vi "Create.vi"(8 "error in (no error)":errorcluster, 9 "Calculation Period (ms)":u32=500, 10 "XNET Session":refnum<k21>, 11 "LINBus_Load_Calculator in":refnum<class "LINBus_Load_Calculator.lvclass">) -> (0 "error out":errorcluster, 3 "LINBus_Load_Calculator out":refnum<class "LINBus_Load_Calculator.lvclass">)   [LabVIEW 2019, in "XNET-Bus-Load-Calculator.lvlib" / "LINBus_Load_Calculator.lvclass"]
uses:
  LINBus_Load_Calculator.lvclass
  GenBus/GenBus_Load_Calculator.lvclass
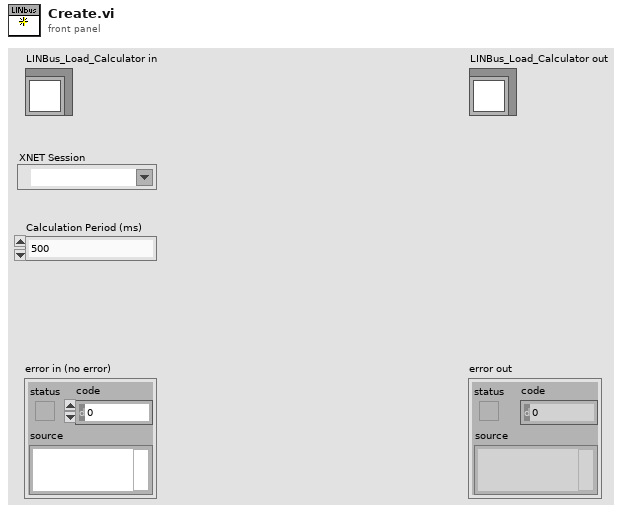
[diagram p1: front panel]
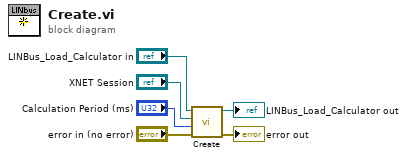
[diagram p0: block diagram]
diagram:
  n1 = call-parent "Create.vi"("error in (no error)"="error in (no error)", "Calculation Period (ms)"="Calculation Period (ms)", "XNET Session"="XNET Session", "GenBus_Load_Calculator in"="LINBus_Load_Calculator in") -> ("error out"=→"error out":errorcluster, "GenBus_Load_Calculator out"=→"LINBus_Load_Calculator out":refnum<class "LINBus_Load_Calculator.lvclass">)  [unwired: 6 in]
